vi "getNumChannels.vi"(8 "error in (no error)":errorcluster, 11 "DAQ in":refnum<class "DAQ.lvclass">) -> (0 "error out":errorcluster, 2 "NumChannels":i32, 3 "DAQ out":refnum<class "DAQ.lvclass">)   [LabVIEW 2016, in "DAQ.lvclass"]
uses:
  DAQ.lvclass
  DAQ.lvclass/DAQ.ctl
  <vilib>/regexp/Match Regular Expression.xnode
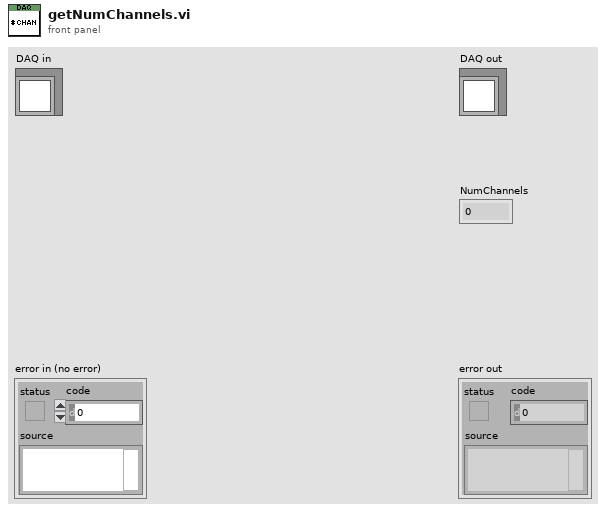
[diagram p1: front panel]
types:
  T1 = typedef "DAQ.lvclass/PrivateEvents--DAQ.AI.Channels.ctl" = string
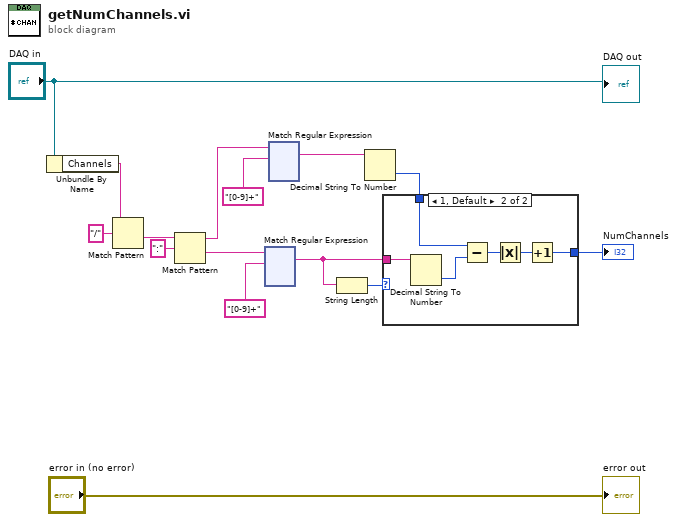
[diagram p0: block diagram]
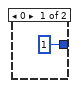
[diagram p2: hidden frame]
diagram:
  n1 = Unbundle By Name("DAQ in") -> ("Channels"=w2:T1)
  n2 = Match Pattern(string=w2, regular expression="/") -> (after substring=w6:T1)  [unwired: 1 in, 3 out]
  n3 = Match Pattern(string=w6, regular expression=":") -> (before substring=w11:T1, after substring=w10:T1)  [unwired: 1 in, 2 out]
  n4 = xnode "Match Regular Expression"("input string"=w10, "regular expression"="[0-9]+") -> ("whole match"=w13:string)  [unwired: 4 in, 4 out]
  n5 = xnode "Match Regular Expression"("input string"=w11, "regular expression"="[0-9]+") -> ("whole match"=w8:string)  [unwired: 4 in, 4 out]
  n6 = String Length(string=w13) -> (length=w14:i32)
  n7 = Decimal String To Number(string=w8) -> (number=w9:i32)  [unwired: 2 in, 1 out]
  n8 = case shown="1, Default" w14 {
    tunnel: w9 -> [_ w22]
    tunnel: [1 w18] -> w15
    tunnel: w13 -> [_ w17]
    frame 0 {
    }
    frame 1, Default {
      n9 = Decimal String To Number(string=w17) -> (number=w21:i32)  [unwired: 2 in, 1 out]
      n10 = Subtract(x=w22, y=w21) -> (x-y=w20:i32)
      n11 = Absolute Value(x=w20) -> (abs(x)=w19:i32)
      n12 = Increment(x=w19) -> (x+1=w18:i32)
    }
  }
  "NumChannels" <- w15
  "error out" <- "error in (no error)"
  "DAQ out" <- "DAQ in"
